vi "Test Suite Method Name Qualified.vi"(8 "error in (no error)":errorcluster, 11 "Test Case In":refnum<class "LUnit Test Suite Tests.lvclass">) -> (0 "error out":errorcluster, 3 "Test Case Out":refnum<class "LUnit Test Suite Tests.lvclass">)   [LabVIEW 2020, in "LUnit Test Suite Tests.lvclass"]
uses:
  LUnit Test Suite Tests.lvclass
  C:/Program Files (x86)/National Instruments/LabVIEW 2020/vi.lib/Astemes/LUnit/Test Case.lvclass
  Core/Result/Result.ctl
  Core/Result/Status.ctl
  Core/Result/Type.ctl
  Test Case Test Double/Test Case Test Double.lvclass
  C:/git/astemes-lunit/source/Core/LUnit Test Case/LUnit Test Case.lvclass
  <vilib>/Astemes/LUnit/Test Case.lvclass/Test Case.ctl
  <vilib>/Astemes/LUnit/Set Assertion Type.vi
  <vilib>/Astemes/LUnit/Palette/Pass.vi
  <vilib>/Astemes/LUnit/Palette/Fail.vi
  <vilib>/Astemes/LUnit/Add test result.vi
  <vilib>/Astemes/LUnit/LUnit Record Assertion Result.vi
  <vilib>/Astemes/LUnit/LUnit Aggregate Assertion Results.vi
  <vilib>/Astemes/LUnit/Method Result/LUnit Merge Status.vi
  <vilib>/Astemes/LUnit/LUnit Concatenate result strings.vi
  Mock Result Observer/Mock Result Observer.lvclass
  C:/git/astemes-lunit/source/Core/Result Observer/Result Observer.lvclass
  Core/LUnit Test Suite/LUnit Test Suite.lvclass
  <vilib>/Astemes/LUnit/Test Case.lvclass
  Core/Result/Result.lvlib
panel:
  out "Results":T1[](array[typedef])
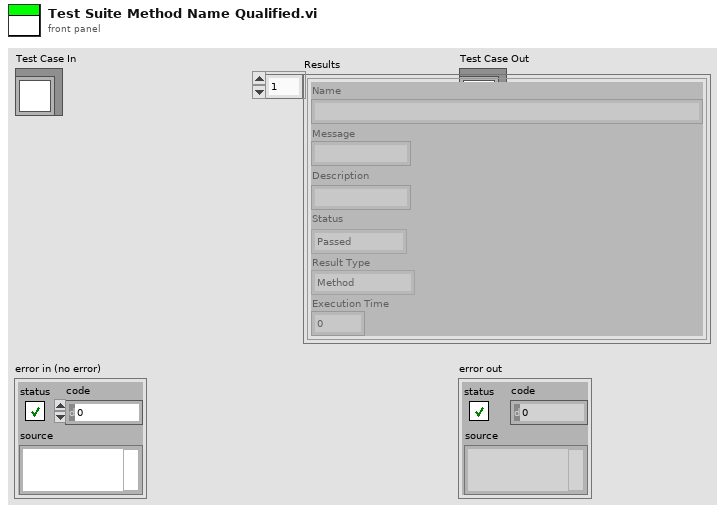
[diagram p1: front panel]
types:
  T1 = typedef "Result.lvlib/Result.ctl" = cluster{"Name":string, "Message":string, "Description":string, "Status":T2, "Result Type":T3, "Execution Time":dbl}
  T2 = typedef "Result.lvlib/Status.ctl" = enum16{"", "Passed", "Failed", "Error", "Skipped", "Setup Error", "Broken", "Teardown Error"}
  T3 = typedef "Result.lvlib/Type.ctl" = enum16{"Method", "Case", "Suite", "Pass", "Fail", "Skip", "Pass if", "Fail if", "Pass if Error", "Fail if Error", "Pass if Equal", "Fail if Equal"}
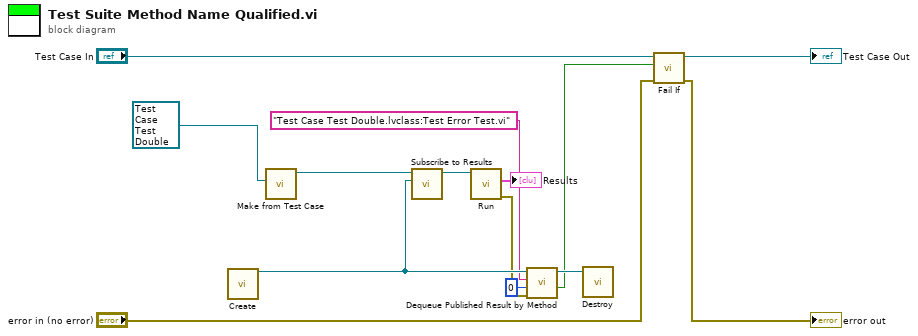
[diagram p0: block diagram]
diagram:
  n1 = call "Create.vi"() -> ("Mock Result Observer out"=w6:refnum<class "Mock Result Observer.lvclass">)  [unwired: 10 in, 1 out]
  n2 = call "Make from Test Case.vi"("LUnit Test Case"=refnum<class "Test Case Test Double.lvclass"> refnum ("LUnit Test Case V2 Test Double.lvclass")) -> ("LUnit Test Suite Out"=w10:refnum<class "LUnit Test Suite.lvclass">)  [unwired: 9 in, 1 out]
  n3 = call-dynamic "Subscribe to Results.vi"("Result Observer"=w6, "LUnit Test Suite In"=w10) -> ("LUnit Test Suite Out"=w7:refnum<class "LUnit Test Suite.lvclass">)  [unwired: 8 in, 1 out]
  n4 = call-dynamic "Run.vi"("LUnit Test Suite In"=w7) -> ("error out"=w5:errorcluster, "Results"=→"Results":T1[])  [unwired: 9 in]
  n5 = call "Dequeue Published Result by Method.vi"("error in (no error)"=w5, "timeout in ms"=0, "Method Name"="Test Case Test Double.lvclass:Test Error Test.vi", "Mock Result Observer In"=w6) -> ("timed out?"=w2:bool, "Mock Result Observer Out"=w4:refnum<class "Mock Result Observer.lvclass">)  [unwired: 4 in, 2 out]
  n6 = call "Destroy.vi"("Mock Result Observer in"=w4) -> ()  [unwired: 9 in, 2 out]
  n7 = call <vilib>:"Fail If.vi"("error in (no error)"="error in (no error)", "Fail?"=w2, "LUnit Test Case In"="Test Case In") -> ("error out"=→"error out":errorcluster, "LUnit Test Case Out"=→"Test Case Out":refnum<class "LUnit Test Suite Tests.lvclass">)  [unwired: 7 in]
